vi "Stop Core.vi"(10 "final error code":i32, 11 "Sensor in":refnum<class "Sensor.lvclass">) -> (3 "Sensor out":refnum<class "Sensor.lvclass">)   [LabVIEW 2012, in "Sensor Definition.lvlib" / "Sensor.lvclass"]
doc: "(<B>Filename</B>: Actor Framework.lvlib:Actor.lvclass:Stop Core.vi)\n\nDefines what the actor does before it stops. Use the <B>final error code</B> input to determine whether the actor shut down in response to an error.\n\nBy default, this method does nothing. A descendant class may override it to define behavior, such as shutting down any processes the actor initiated in its override of the Actor Core method."
uses:
  Sensor.lvclass
  <vilib>/ActorFramework/Time-Delayed Send Message/Time-Delay Override Options.ctl
  <vilib>/ActorFramework/Actor/Actor.lvclass/Actor.ctl
  <vilib>/ActorFramework/Message Enqueuer/Message Enqueuer.lvclass/Message Enqueuer.ctl
  Sensor.lvclass/Sensor.ctl
  <vilib>/ActorFramework/Actor/Actor.lvclass
  DemoMain Messages/Remove Sensor Msg/Remove Sensor Msg.lvclass/Remove Sensor Msg.ctl
  Read Listening SensorViews.vi
  Read Scheduled Delivery Notifier.vi
  <vilib>/ActorFramework/Message Enqueuer/Init from Existing Queue.vi
  <vilib>/ActorFramework/Message Enqueuer/Enqueue.vi
  <vilib>/ActorFramework/Message Priority Queue/Priority Enqueue.vi
  <vilib>/ActorFramework/Message Enqueuer/Message Enqueuer.lvclass
  DemoMain Messages/Remove Sensor Msg/Remove Sensor Msg.lvclass
  <vilib>/ActorFramework/Stop Msg/Stop Msg.lvclass
  Win8uiFramework/Win8uiFramework.lvlib
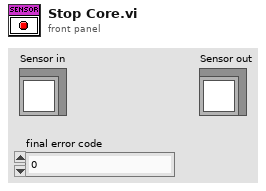
[diagram p1: front panel]
types:
  T1 = typedef "Time-Delay Override Options.ctl" = enum16{"Send next copy now", "Skip next scheduled copy", "Send next copy now and stop all further copies", "Stop all further copies"}
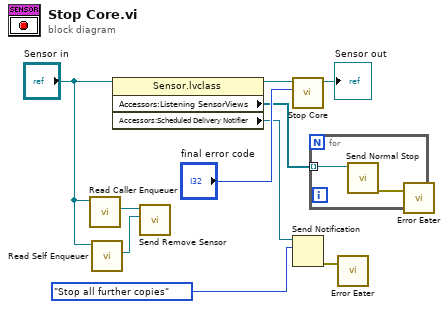
[diagram p0: block diagram]
diagram:
  n1 = call <vilib>:"Read Caller Enqueuer.vi"("Actor"="Sensor in") -> ("Caller Enqueuer"=w3:refnum<class "Message Enqueuer.lvclass">)  [unwired: 10 in]
  n2 = call <vilib>:"Read Self Enqueuer.vi"("Actor"="Sensor in") -> ("Self Enqueuer"=w2:refnum<class "Message Enqueuer.lvclass">)  [unwired: 10 in]
  n3 = property class="Sensor.lvclass"(reference="Sensor in") -> (reference out=w8:refnum<class "Sensor.lvclass">, "Accessors:Listening SensorViews"=w7:refnum<class "Message Enqueuer.lvclass">[], "Accessors:Scheduled Delivery Notifier"=w6:refnum<notifier>)  [unwired: 1 in, 1 out]
  n4 = call "Send Remove Sensor.vi"("Sensor Enqueuer"=w2, "Message Enqueuer"=w3) -> ()  [unwired: 8 in, 2 out]
  n5 = call-parent "Stop Core.vi"("final error code"="final error code", "Actor in"=w8) -> ("Actor out"=→"Sensor out":refnum<class "Sensor.lvclass">)  [unwired: 9 in]
  n6 = Send Notification(notification=Time-Delay_Override_Options."Stop all further copies", notifier=w6) -> (error out=w4:errorcluster)  [unwired: 1 in, 1 out]
  n7 = for {
    tunnel: w7 -> [w12] mode=indexing
    n8 = call <vilib>:"Send Normal Stop.vi"("Message Enqueuer"=w12) -> ("error out"=w11:errorcluster)  [unwired: 10 in]
    n9 = call "Error Eater.vi"("error in (no error)"=w11) -> ()  [unwired: 2 in]
  }
  n10 = call "Error Eater.vi"("error in (no error)"=w4) -> ()  [unwired: 2 in]
